vi "Alle_Kanten_aller_Lichtgitter.vi"(8 "Fehler in":errorcluster, 11 "Cluster in":T1={"Initialisierung"={"Online?"=FALSE, "Grundpfad"=path "", "Kamera Oben"="", "IP-Adresse Flüssiglinse"="", "Flüssiglinse"=refnum, "Kamera Unten"="", "IP-Adresse SPS"="", "SPS-Verbindung"={"TCP Connection Ref"=refnum, "IP address"="", "timeout ms"=5000, "Connected?"=FALSE, "PLC Type"=enum."S7 1200", "Rack S7 400"=0, "Slot S7 400"=0, "PDU Size"=0, "connection semaphore"=refnum}, "IP-Adresse Lichtgitter"="", "Lichtgitter"=refnum, "Skalierungsfaktor"=0.0, "Bilder Oben"=[], "Bild Unten"=refnum, "Bild Ausschnitt Unten"=refnum}, "Einstellungen"={"Gesamtablauf gestartet"=FALSE, "i. O. Bilder speichern"=FALSE, "Bildspeicherung Offline"=FALSE, "Ausgewähltes Offline-Datum"="", "Ausgewähltes Offline-Teil"="", "Speicherpfad Bilder"=path ""}, "Artikeldaten"={"Artikelnummer"="", "Fertigungsauftrag"="", "Muster ISO"=refnum, "Belichtungszeit Referenzmarken"=0.0, "Fokus Referenzmarken"=0.0, "Belichtungszeit ISO"=0.0, "Fokus ISO"=0.0, "Belichtungszeit Unten"=0.0, "Kontaktanzahl"=0, "Aktueller Kontakt"=0, "Kontaktposition"={"x"=0.0, "y"=0.0}, "ISO-Muster nicht vorhanden"=FALSE, "Winkel ISO"=0.0, "Mittelpunkt ISO"={"x"=0.0, "y"=0.0}}, "Werte Kamera Oben"={"Koordinatensystem"={"Punkt x-Achse"={"X"=0.0, "Y"=0.0}, "Ursprung"={"X"=0.0, "Y"=0.0}, "Punkt y-Achse"={"X"=0.0, "Y"=0.0}}, "Position Kontakt"={"x"=0.0, "y"=0.0}, "Durchmesser Loch"=0.0, "Winkel Kontakt"=0.0, "Position Kontakt umgerechnet"={"x"=0.0, "y"=0.0}}, "Werte Kamera Unten"={"Prüfung Unten n. i. O."=FALSE}, "Werte Lichtgitter"={"Messwerte Referenzmarken"=[], "Mittelpunkt Referenzmarken"={"x"=0.0, "y"=0.0}, "Messwerte Kontakt"=[], "Offset"={"x"=0.0, "y"=0.0}}, "Rückmeldungen"={"Koordinaten ermittelt"=FALSE, "Vermessung Lichtgitter fertig"=FALSE, "Nachkontrolle Kamera Unten fertig"=FALSE}, "Fehler"={"Referenzen nicht gefunden"=FALSE, "Kontakt nicht gefunden"=FALSE, "Referenzen nicht in Lichtgitter"=FALSE, "Kontakt zu groß"=FALSE, "Kontakt zu klein"=FALSE}, "Statistik"={"Statistiken"=[]}, "Timer"={"Timer Start Position"=0, "Timer Start Lichtgitter"=0, "Timer Start Kamera Unten"=0}}) -> (0 "Fehler out":errorcluster, 1 "Anzahl Kanten":i32[](array[numeric]), 2 "Lese- und Schreibestrings":string, 3 "Cluster out":T1={"Initialisierung"={"Online?"=FALSE, "Grundpfad"=path "", "Kamera Oben"="", "IP-Adresse Flüssiglinse"="", "Flüssiglinse"=refnum, "Kamera Unten"="", "IP-Adresse SPS"="", "SPS-Verbindung"={"TCP Connection Ref"=refnum, "IP address"="", "timeout ms"=5000, "Connected?"=FALSE, "PLC Type"=enum."S7 1200", "Rack S7 400"=0, "Slot S7 400"=0, "PDU Size"=0, "connection semaphore"=refnum}, "IP-Adresse Lichtgitter"="", "Lichtgitter"=refnum, "Skalierungsfaktor"=0.0, "Bilder Oben"=[], "Bild Unten"=refnum, "Bild Ausschnitt Unten"=refnum}, "Einstellungen"={"Gesamtablauf gestartet"=FALSE, "i. O. Bilder speichern"=FALSE, "Bildspeicherung Offline"=FALSE, "Ausgewähltes Offline-Datum"="", "Ausgewähltes Offline-Teil"="", "Speicherpfad Bilder"=path ""}, "Artikeldaten"={"Artikelnummer"="", "Fertigungsauftrag"="", "Muster ISO"=refnum, "Belichtungszeit Referenzmarken"=0.0, "Fokus Referenzmarken"=0.0, "Belichtungszeit ISO"=0.0, "Fokus ISO"=0.0, "Belichtungszeit Unten"=0.0, "Kontaktanzahl"=0, "Aktueller Kontakt"=0, "Kontaktposition"={"x"=0.0, "y"=0.0}, "ISO-Muster nicht vorhanden"=FALSE, "Winkel ISO"=0.0, "Mittelpunkt ISO"={"x"=0.0, "y"=0.0}}, "Werte Kamera Oben"={"Koordinatensystem"={"Punkt x-Achse"={"X"=0.0, "Y"=0.0}, "Ursprung"={"X"=0.0, "Y"=0.0}, "Punkt y-Achse"={"X"=0.0, "Y"=0.0}}, "Position Kontakt"={"x"=0.0, "y"=0.0}, "Durchmesser Loch"=0.0, "Winkel Kontakt"=0.0, "Position Kontakt umgerechnet"={"x"=0.0, "y"=0.0}}, "Werte Kamera Unten"={"Prüfung Unten n. i. O."=FALSE}, "Werte Lichtgitter"={"Messwerte Referenzmarken"=[], "Mittelpunkt Referenzmarken"={"x"=0.0, "y"=0.0}, "Messwerte Kontakt"=[], "Offset"={"x"=0.0, "y"=0.0}}, "Rückmeldungen"={"Koordinaten ermittelt"=FALSE, "Vermessung Lichtgitter fertig"=FALSE, "Nachkontrolle Kamera Unten fertig"=FALSE}, "Fehler"={"Referenzen nicht gefunden"=FALSE, "Kontakt nicht gefunden"=FALSE, "Referenzen nicht in Lichtgitter"=FALSE, "Kontakt zu groß"=FALSE, "Kontakt zu klein"=FALSE}, "Statistik"={"Statistiken"=[]}, "Timer"={"Timer Start Position"=0, "Timer Start Lichtgitter"=0, "Timer Start Kamera Unten"=0}})   [LabVIEW 2024]
doc: "Überprüft ob die richtige Anzahl an Kanten in den Lichtgittern vorhanden sind und schreibt alle Messwerte in das Cluster."
uses:
  Typdefinitionen/Cluster.ctl
  <vilib>/userDefined/High Color/IMAQdx.ctl
  <vilib>/DATA AHEAD/SP7/typedefs/S7 Connection.ctl
  <vilib>/DATA AHEAD/SP7/typedefs/PLC Type.ctl
  <vilib>/vision/Image Controls.llb/IMAQ Image.ctl
  Typdefinitionen/Koordinatensystem.ctl
  Typdefinitionen/Statistik.ctl
  <vilib>/Utility/file.llb/Read Delimited Spreadsheet (DBL).vi
  <vilib>/DATA AHEAD/SP7/SP7.lvlib
panel:
  in  "milliseconds to wait":u32=35
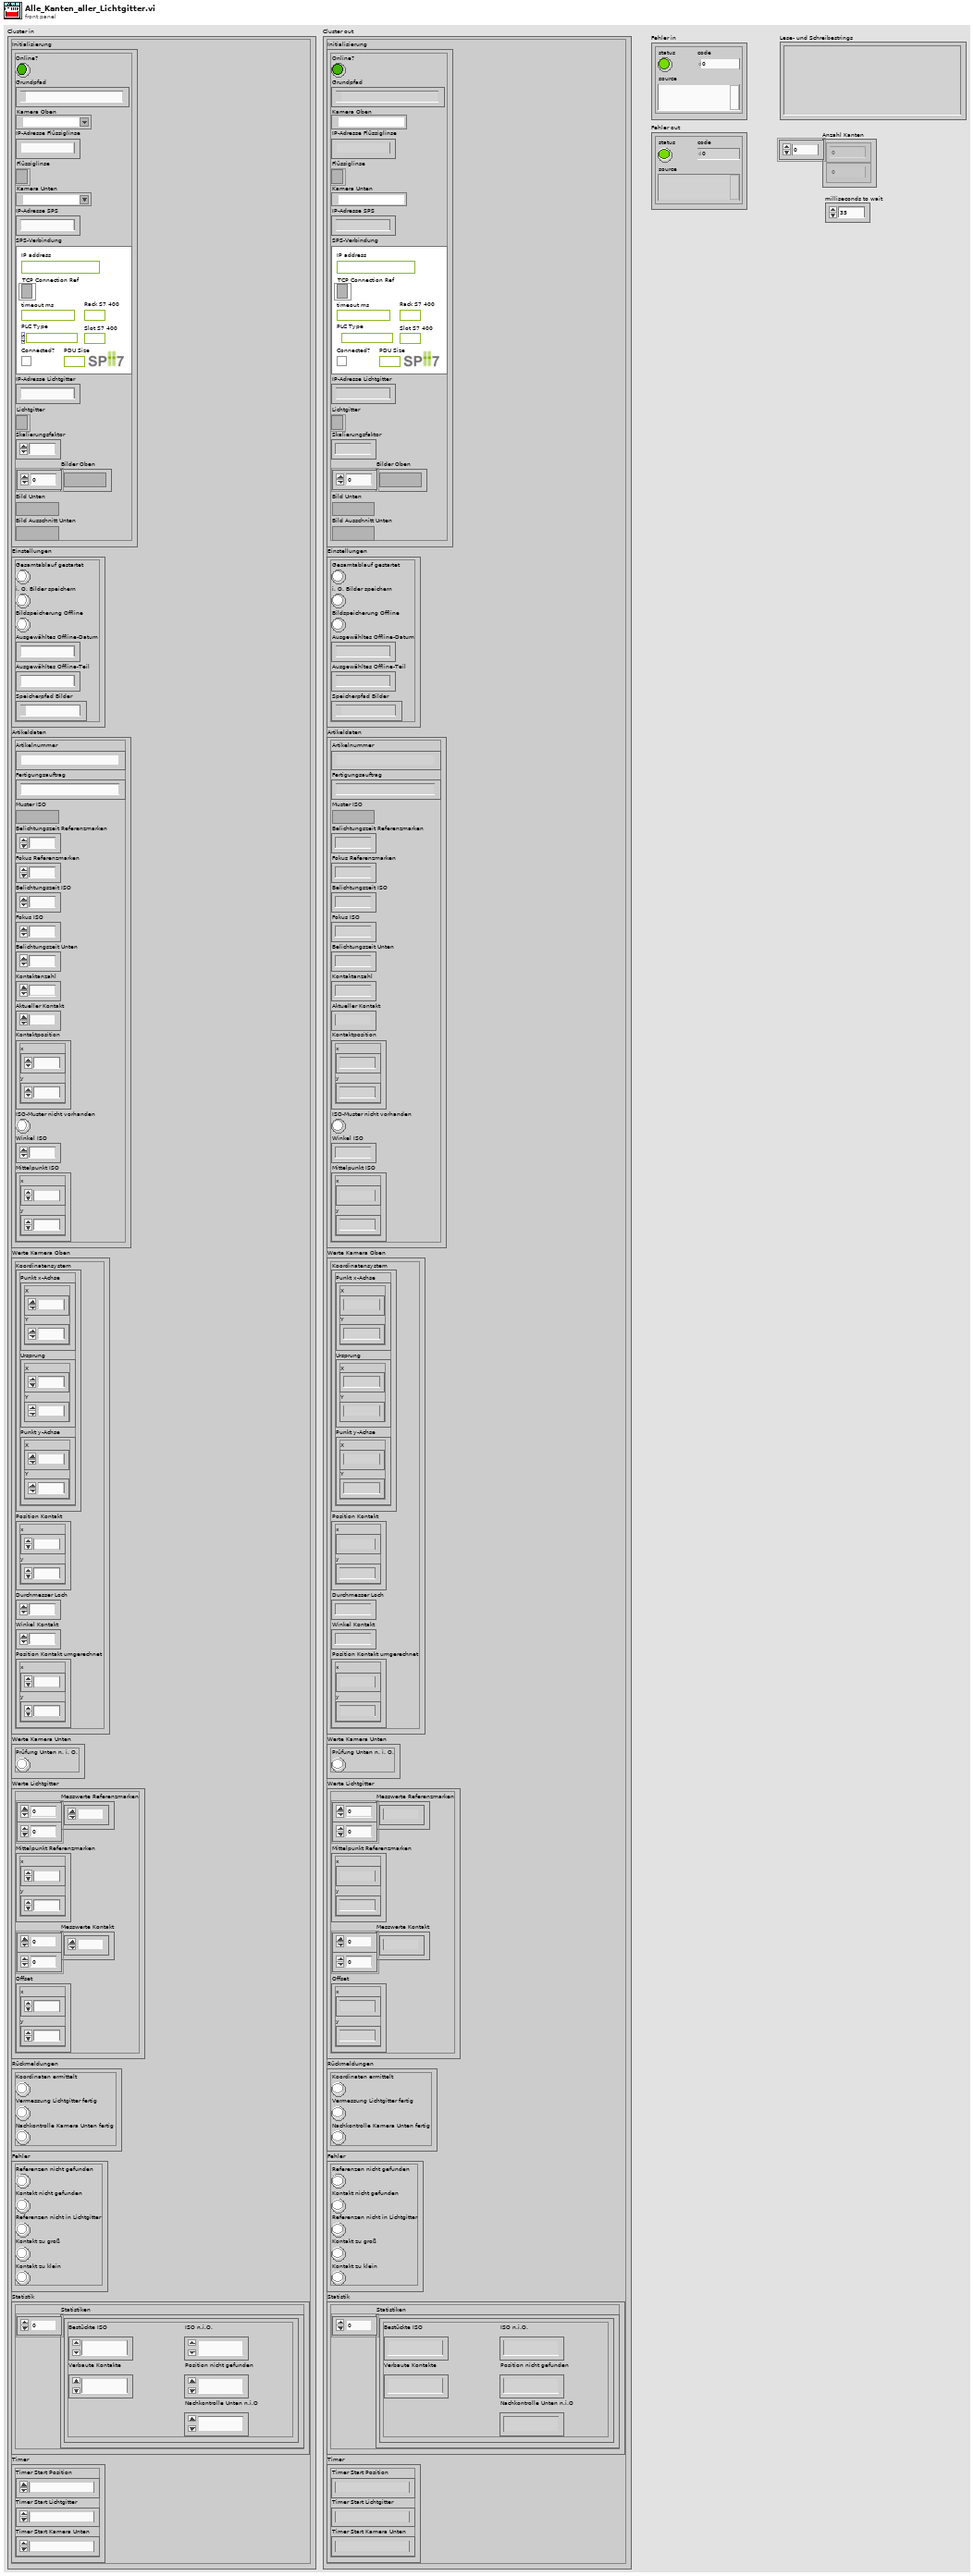
[diagram p1: front panel]
types:
  T1 = typedef "Cluster.ctl" = cluster{"Initialisierung":cluster{"Online?":bool, "Grundpfad":path, "Kamera Oben":T2, "IP-Adresse Flüssiglinse":string, "Flüssiglinse":refnum<k5>, "Kamera Unten":T2, "IP-Adresse SPS":string, "SPS-Verbindung":T3, "IP-Adresse Lichtgitter":string, "Lichtgitter":refnum<k5>, "Skalierungsfaktor":dbl, "Bilder Oben":T6[], "Bild Unten":T6, "Bild Ausschnitt Unten":T6}, "Einstellungen":cluster{"Gesamtablauf gestartet":bool, "i. O. Bilder speichern":bool, "Bildspeicherung Offline":bool, "Ausgewähltes Offline-Datum":string, "Ausgewähltes Offline-Teil":string, "Speicherpfad Bilder":path}, "Artikeldaten":cluster{"Artikelnummer":string, "Fertigungsauftrag":string, "Muster ISO":T6, "Belichtungszeit Referenzmarken":dbl, "Fokus Referenzmarken":dbl, "Belichtungszeit ISO":dbl, "Fokus ISO":dbl, "Belichtungszeit Unten":dbl, "Kontaktanzahl":u32, "Aktueller Kontakt":i16, "Kontaktposition":cluster{"x":sgl, "y":sgl}, "ISO-Muster nicht vorhanden":bool, "Winkel ISO":sgl, "Mittelpunkt ISO":cluster{"x":dbl, "y":dbl}}, "Werte Kamera Oben":cluster{"Koordinatensystem":T7, "Position Kontakt":cluster{"x":dbl, "y":dbl}, "Durchmesser Loch":dbl, "Winkel Kontakt":dbl, "Position Kontakt umgerechnet":cluster{"x":dbl, "y":dbl}}, "Werte Kamera Unten":cluster{"Prüfung Unten n. i. O.":bool}, "Werte Lichtgitter":cluster{"Messwerte Referenzmarken":dbl[][], "Mittelpunkt Referenzmarken":cluster{"x":dbl, "y":dbl}, "Messwerte Kontakt":dbl[][], "Offset":cluster{"x":dbl, "y":dbl}}, "Rückmeldungen":cluster{"Koordinaten ermittelt":bool, "Vermessung Lichtgitter fertig":bool, "Nachkontrolle Kamera Unten fertig":bool}, "Fehler":cluster{"Referenzen nicht gefunden":bool, "Kontakt nicht gefunden":bool, "Referenzen nicht in Lichtgitter":bool, "Kontakt zu groß":bool, "Kontakt zu klein":bool}, "Statistik":cluster{"Statistiken":T8[]}, "Timer":cluster{"Timer Start Position":u32, "Timer Start Lichtgitter":u32, "Timer Start Kamera Unten":u32}}
  T2 = typedef "IMAQdx.ctl" = refnum<k21>
  T3 = typedef "SP7.lvlib/S7 Connection.ctl" = cluster{"TCP Connection Ref":refnum<k5>, "IP address":string, "timeout ms":i32, "Connected?":bool, "PLC Type":T4, "Rack S7 400":u8, "Slot S7 400":u8, "PDU Size":u16, "connection semaphore":T5}
  T4 = typedef "SP7.lvlib/PLC Type.ctl" = enum16{"S7 200", "S7 300/400", "S7 1200", "S7 1500", "LOGO!8"}
  T5 = typedef "Semaphore RefNum" = refnum<k1>
  T6 = typedef "IMAQ Image.ctl" = refnum<image>
  T7 = typedef "Koordinatensystem.ctl" = cluster{"Punkt x-Achse":cluster{"X":sgl, "Y":sgl}, "Ursprung":cluster{"X":sgl, "Y":sgl}, "Punkt y-Achse":cluster{"X":sgl, "Y":sgl}}
  T8 = typedef "Statistik.ctl" = cluster{"Bestückte ISO":u32, "Verbaute Kontakte":u32, "ISO n.i.O.":u32, "Nachkontrolle Unten n.i.O":u32, "Position nicht gefunden":u32}
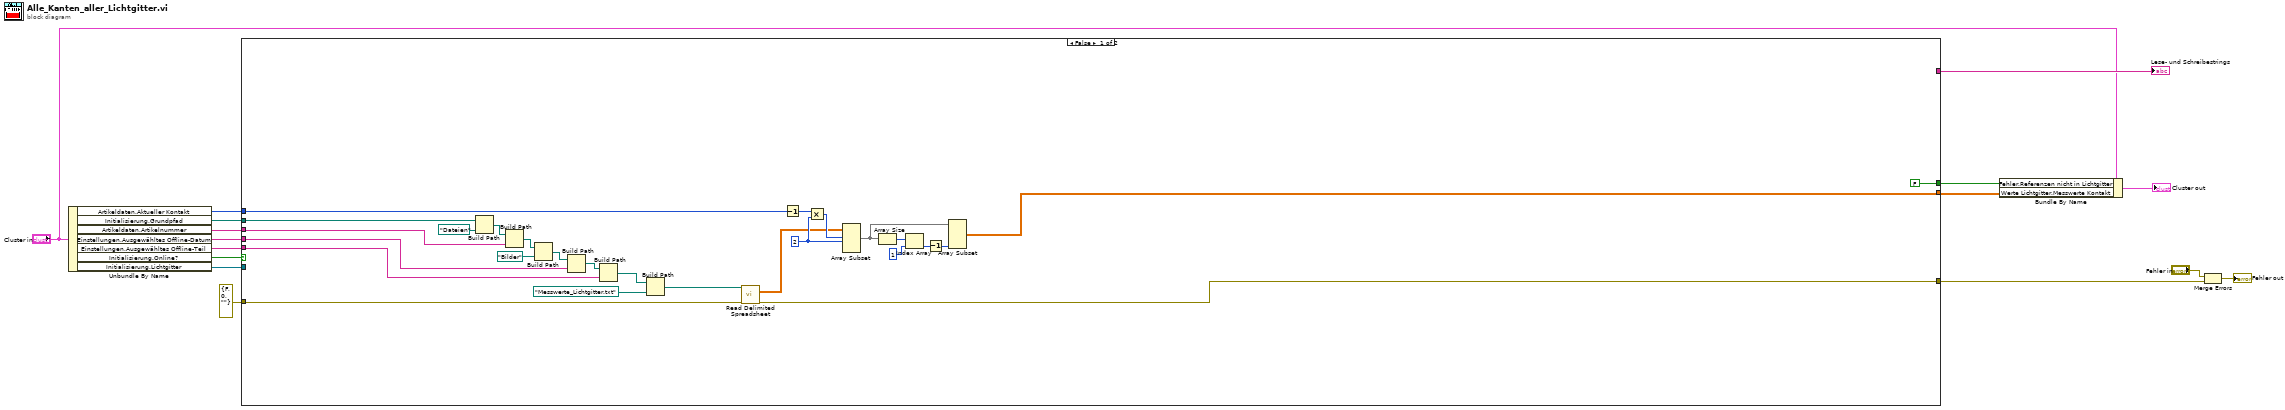
[diagram p0: block diagram]
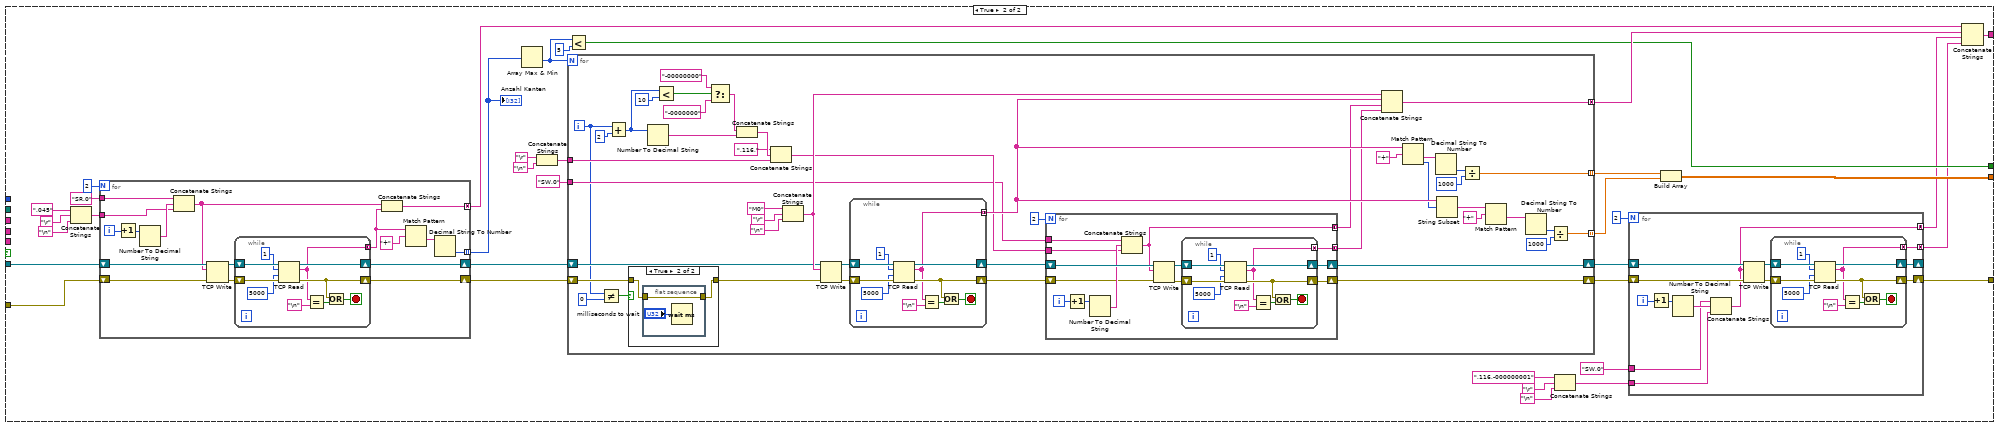
[diagram p2: hidden frame]
diagram:
  n1 = Unbundle By Name("Cluster in") -> ("Artikeldaten.Aktueller Kontakt"=w2:i16, "Initialisierung.Grundpfad"=w5:path, "Artikeldaten.Artikelnummer"=w4:string, "Einstellungen.Ausgewähltes Offline-Datum"=w6:string, "Einstellungen.Ausgewähltes Offline-Teil"=w7:string, "Initialisierung.Online?"=w8:bool, "Initialisierung.Lichtgitter"=w12:refnum<k5>)
  n2 = case shown="False" w8 {
    tunnel: [_ w65] -> w14
    tunnel: [w34 w54] -> w13
    tunnel: w12 -> [_ w60]
    tunnel: [w18 w59] -> w1
    tunnel: [FALSE w58] -> w9
    tunnel: w7 -> [w39 _]
    tunnel: w5 -> [w28 _]
    tunnel: w6 -> [w40 _]
    tunnel: w4 -> [w25 _]
    tunnel: errorcluster {"status"=FALSE, "code"=0, "source"=""} ("Fehler in 2") -> [w35 w57]
    tunnel: w2 -> [w33 _]
    frame False {
      w31 = 2 ("length")
      n3 = Build Path(base path=w28, name or relative path=path "Dateien") -> (appended path=w27:path)
      n4 = Build Path(base path=w27, name or relative path=w25) -> (appended path=w42:path)
      n5 = Build Path(base path=w42, name or relative path=path "Bilder") -> (appended path=w29:path)
      n6 = Build Path(base path=w29, name or relative path=w40) -> (appended path=w41:path)
      n7 = Build Path(base path=w41, name or relative path=w39) -> (appended path=w38:path)
      n8 = Build Path(base path=w38, name or relative path=path "Messwerte_Lichtgitter.txt") -> (appended path=w36:path)
      n9 = call-poly <vilib>:"Read Delimited Spreadsheet.vi"("file path (dialog if empty)"=w36, "error in (no error)"=w35) -> ("all rows"=w17:dbl[][], "error out"=w34:errorcluster)  [unwired: 8 in, 4 out]
      n10 = Decrement(x=w33) -> (x-1=w32:i16)
      n11 = Multiply(x=w32, y=w31) -> (x*y=w30:i32)
      n12 = Array Subset(array=w17, index (row)=w30, length (row)=w31) -> (w19:dbl[][])  [unwired: 2 in]
      n13 = Array Size(array=w19) -> (size(s)=w23:i32[])
      n14 = Index Array(array=w23, index=1) -> (element=w21:i32)
      n15 = Decrement(x=w21) -> (x-1=w20:i32)
      n16 = Array Subset(array=w19, length (col)=w20) -> (w18:dbl[][])  [unwired: 3 in]
    }
    frame True {
      n17 = Concatenate Strings(",045" ("string"), "\r", "\n") -> (w74:string)
      n18 = for {
        N: 2 -> [_]
        tunnel: "SR,0" ("string") -> [w195]
        shift-right: [w198] -> w69
        shift-left: w60 -> [w196]
        shift-right: [w197] -> w73
        shift-left: w57 -> [w192]
        tunnel: w74 -> [w193]
        tunnel: [w190] -> w66 mode=concatenating
        tunnel: [w186] -> w63 mode=indexing
        i -> [w200]
        n19 = Increment(x=w200) -> (x+1=w199:i32)
        n20 = Number To Decimal String(number=w199) -> (decimal integer string=w194:string)  [unwired: 1 in]
        n21 = Concatenate Strings(w195, w194, w193) -> (w191:string)
        n22 = TCP Write(connection ID=w196, data in=w191, error in (no error)=w192) -> (connection ID out=w201:refnum<k5>, error out=w202:errorcluster)  [unwired: 1 in, 1 out]
        n23 = while {
          shift-right: [w210] -> w198
          shift-left: w201 -> [w212]
          shift-right: [w206] -> w197
          shift-left: w202 -> [w211]
          tunnel: [w203] -> w187 mode=concatenating
          stop <- w205 stop-if-true
          n24 = TCP Read(connection ID=w212, bytes to read=1, error in (no error)=w211, 9:5000 ("timeout ms (25000)")) -> (connection ID out=w210:refnum<k5>, data out=w203:string, error out=w206:errorcluster)  [unwired: 1 in]
          n25 = Equal?(x=w203, y="\n") -> (x = y?=w207:bool)
          n26 = Or(x=w206, y=w207) -> (x .or. y?=w205:bool)
        }
        n27 = Concatenate Strings(w191, w187) -> (w190:string)
        n28 = Match Pattern(string=w187, regular expression="+" ("search string")) -> (after substring=w189:string)  [unwired: 1 in, 3 out]
        n29 = Decimal String To Number(string=w189) -> (number=w186:i32)  [unwired: 2 in, 1 out]
      }
      "Anzahl Kanten" <- w63
      n30 = Array Max & Min(array=w63) -> (min value=w45:i32)  [unwired: 3 out]
      n31 = Concatenate Strings("\r", "\n") -> (w70:string)
      n32 = for {
        N: w45 -> [_]
        shift-right: [w112] -> w56
        shift-left: w69 -> [w117]
        shift-right: [w111] -> w55
        shift-left: w73 -> [w118]
        tunnel: w70 -> [w147]
        tunnel: [w143] -> w67 mode=concatenating
        tunnel: [w121] -> w61 mode=indexing
        tunnel: "SW,0" ("string") -> [w107]
        tunnel: [w120] -> w62 mode=indexing
        i -> [w104]
        n33 = Not Equal?(x=w104, y=0) -> (x != y?=w109:bool)
        n34 = Add(x=w104, y=2) -> (x+y=w103:i32)
        n35 = case shown="True" w109 {
          tunnel: w118 -> [w148 w150]
          tunnel: [w148 w149] -> w116
          frame False {
          }
          frame True {
            n36 = flat-sequence {
              tunnel: w150 -> [w152]
              tunnel: [w152] -> w149
              frame #0 {
                n37 = Wait (ms)(milliseconds to wait="milliseconds to wait") -> ()  [unwired: 1 out]
              }
            }
          }
        }
        n38 = Number To Decimal String(number=w103) -> (decimal integer string=w146:string)  [unwired: 1 in]
        n39 = Less?(x=w103, y=10) -> (x < y?=w141:bool)
        n40 = Select(t="-00000000" ("string"), s=w141, f="-0000000" ("string")) -> (s? t:f=w138:string)
        n41 = Concatenate Strings(w138, w146) -> (w145:string)
        n42 = Concatenate Strings(",116," ("string"), w145, w147) -> (w108:string)
        n43 = Concatenate Strings("M0" ("string"), "\r", "\n") -> (w135:string)
        n44 = TCP Write(connection ID=w117, data in=w135, error in (no error)=w116) -> (connection ID out=w132:refnum<k5>, error out=w133:errorcluster)  [unwired: 1 in, 1 out]
        n45 = while {
          shift-right: [w183] -> w113
          shift-left: w132 -> [w185]
          shift-right: [w179] -> w114
          shift-left: w133 -> [w184]
          tunnel: [w176] -> w122 mode=concatenating
          stop <- w178 stop-if-true
          n46 = TCP Read(connection ID=w185, bytes to read=1, error in (no error)=w184, 9:5000 ("timeout ms (25000)")) -> (connection ID out=w183:refnum<k5>, data out=w176:string, error out=w179:errorcluster)  [unwired: 1 in]
          n47 = Equal?(x=w176, y="\n") -> (x = y?=w180:bool)
          n48 = Or(x=w179, y=w180) -> (x .or. y?=w178:bool)
        }
        n49 = for {
          N: 2 -> [_]
          tunnel: w107 -> [w158]
          shift-right: [w161] -> w112
          shift-left: w113 -> [w159]
          shift-right: [w160] -> w111
          shift-left: w114 -> [w155]
          tunnel: w108 -> [w156]
          tunnel: [w154] -> w106 mode=concatenating
          tunnel: [w153] -> w105 mode=concatenating
          i -> [w163]
          n50 = Increment(x=w163) -> (x+1=w162:i32)
          n51 = Number To Decimal String(number=w162) -> (decimal integer string=w157:string)  [unwired: 1 in]
          n52 = Concatenate Strings(w158, w157, w156) -> (w153:string)
          n53 = TCP Write(connection ID=w159, data in=w153, error in (no error)=w155) -> (connection ID out=w164:refnum<k5>, error out=w165:errorcluster)  [unwired: 1 in, 1 out]
          n54 = while {
            shift-right: [w173] -> w161
            shift-left: w164 -> [w175]
            shift-right: [w169] -> w160
            shift-left: w165 -> [w174]
            tunnel: [w166] -> w154 mode=concatenating
            stop <- w168 stop-if-true
            n55 = TCP Read(connection ID=w175, bytes to read=1, error in (no error)=w174, 9:5000 ("timeout ms (25000)")) -> (connection ID out=w173:refnum<k5>, data out=w166:string, error out=w169:errorcluster)  [unwired: 1 in]
            n56 = Equal?(x=w166, y="\n") -> (x = y?=w170:bool)
            n57 = Or(x=w169, y=w170) -> (x .or. y?=w168:bool)
          }
        }
        n58 = Concatenate Strings(w135, w122, w105, w106) -> (w143:string)
        n59 = Match Pattern(string=w122, regular expression="+") -> (after substring=w130:string, offset past match=w119:i32)  [unwired: 1 in, 2 out]
        n60 = Decimal String To Number(string=w130) -> (number=w131:i32)  [unwired: 2 in, 1 out]
        n61 = String Subset(string=w122, offset (0)=w119) -> (substring=w127:string)  [unwired: 1 in]
        n62 = Divide(x=w131, y=1000) -> (x/y=w120:dbl)
        n63 = Match Pattern(string=w127, regular expression="+") -> (after substring=w123:string)  [unwired: 1 in, 3 out]
        n64 = Decimal String To Number(string=w123) -> (number=w124:i32)  [unwired: 2 in, 1 out]
        n65 = Divide(x=w124, y=1000) -> (x/y=w121:dbl)
      }
      n66 = Less?(x=w45, y=5 ("x")) -> (x < y?=w58:bool)
      n67 = Concatenate Strings(",116,-000000001" ("string"), "\r", "\n") -> (w49:string)
      n68 = for {
        N: 2 -> [_]
        shift-right: [w87] -> _
        shift-left: w56 -> [w85]
        shift-right: [w86] -> w54
        shift-left: w55 -> [w83]
        tunnel: [w82] -> w47 mode=concatenating
        tunnel: [w81] -> w48 mode=concatenating
        tunnel: "SW,0" ("string") -> [w80]
        tunnel: w49 -> [w79]
        i -> [w89]
        n69 = Increment(x=w89) -> (x+1=w88:i32)
        n70 = Number To Decimal String(number=w88) -> (decimal integer string=w84:string)  [unwired: 1 in]
        n71 = Concatenate Strings(w80, w84, w79) -> (w81:string)
        n72 = TCP Write(connection ID=w85, data in=w81, error in (no error)=w83) -> (connection ID out=w90:refnum<k5>, error out=w91:errorcluster)  [unwired: 1 in, 1 out]
        n73 = while {
          shift-right: [w99] -> w87
          shift-left: w90 -> [w101]
          shift-right: [w95] -> w86
          shift-left: w91 -> [w100]
          tunnel: [w92] -> w82 mode=concatenating
          stop <- w94 stop-if-true
          n74 = TCP Read(connection ID=w101, bytes to read=1, error in (no error)=w100, 9:5000 ("timeout ms (25000)")) -> (connection ID out=w99:refnum<k5>, data out=w92:string, error out=w95:errorcluster)  [unwired: 1 in]
          n75 = Equal?(x=w92, y="\n") -> (x = y?=w96:bool)
          n76 = Or(x=w95, y=w96) -> (x .or. y?=w94:bool)
        }
      }
      n77 = Build Array(w62, w61) -> (w59:dbl[][])
      n78 = Concatenate Strings(w66, w67, w48, w47) -> (w65:string)
    }
  }
  "Lese- und Schreibestrings" <- w14
  n79 = Bundle By Name(cluster="Cluster in", "Fehler.Referenzen nicht in Lichtgitter"=w9, "Werte Lichtgitter.Messwerte Kontakt"=w1) -> (→"Cluster out":T1)
  n80 = Merge Errors("Fehler in", w13) -> (→"Fehler out":errorcluster)
